vi "turnOppositeToEnemy.vi"(0 "KickToSkill in":refnum<class "KickToSkill.lvclass">, 5 "BallRef":refnum<class "Ball.lvclass">, 7 "Robot":refnum<class "Robot.lvclass">, 9 "EnemyRobotRef":refnum<class "Robot.lvclass">[](array[class]), 11 "error in (no error)":errorcluster) -> (4 "KickToSkill out":refnum<class "KickToSkill.lvclass">, 6 "state out":T1=enum."Farthest", 15 "error out":errorcluster)   [LabVIEW 2020, in "KickToSkill.lvclass"]
uses:
  KickToSkill.lvclass
  Robot_class/Robot.lvclass
  C:/Users/anton/Desktop/RoboIME/SSL_COMP/SSL_AI/Object_class/Object.lvclass
  Ball_class/Ball.lvclass
  turnOppositeToEnemyStates.ctl
  Object_class/Object.lvclass/Object.ctl
  Robot_class/Robot.lvclass/Robot.ctl
  <vilib>/Analysis/baseanly.llb/Real Dot Product.vi
  Object_class/Read x.vi
  Object_class/Read y.vi
  Robot_class/Read dest_orientation.vi
  Utilities_class/Utilities.lvclass
  <vilib>/Analysis/NI_AALBase.lvlib
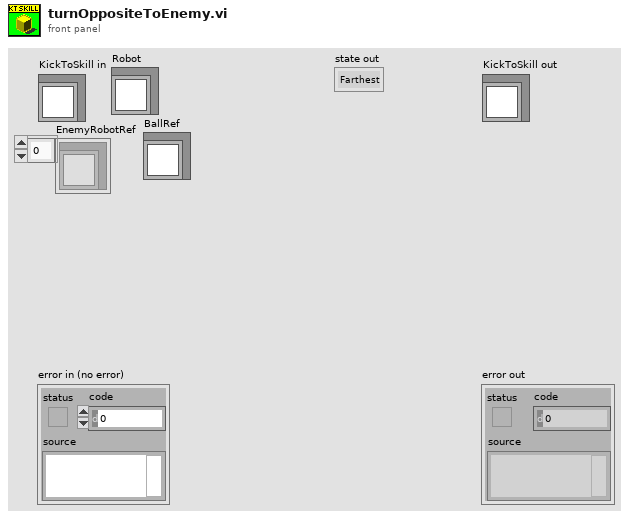
[diagram p1: front panel]
types:
  T1 = typedef "turnOppositeToEnemyStates.ctl" = enum16{"None", "Closest", "Farthest"}
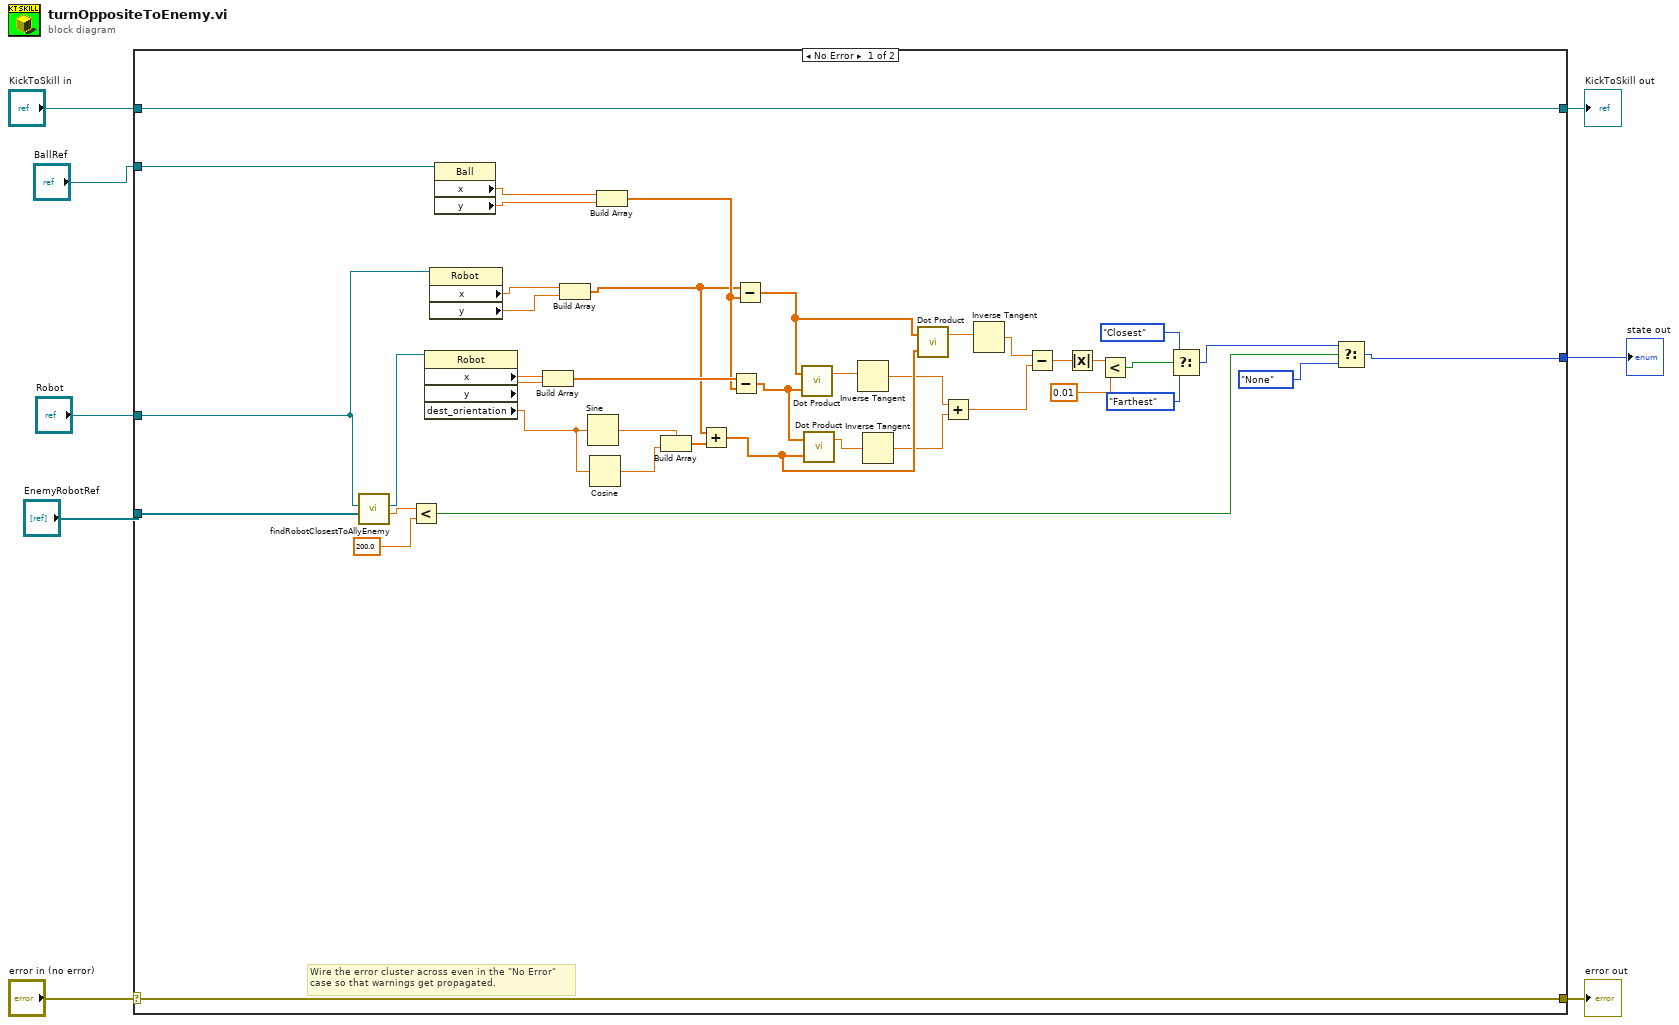
[diagram p0: block diagram]
diagram:
  n1 = case shown="No Error" "error in (no error)" {
    selector: "error in (no error)" -> [w48 w51]
    tunnel: [w48 w51] -> w7
    tunnel: [w49 w50] -> w5
    tunnel: "KickToSkill in" -> [w49 w50]
    tunnel: "EnemyRobotRef" -> [w47 _]
    tunnel: "Robot" -> [w44 _]
    tunnel: "BallRef" -> [w38 _]
    tunnel: [w9 _] -> w1
    frame No Error {
      # "Wire the error cluster across even in the \"No Error\"\ncase so that warnings get propagated."
      n2 = call "findRobotClosestToAllyEnemy.vi"("Ally/Enemy Robots"=w47, "Robot Target"=w44) -> ("Robot distance to other one"=w46:dbl, "Robot"=w43:refnum<class "Robot.lvclass">)  [unwired: 6 in, 2 out]
      n3 = Less?(x=w46, y=200.0 ("Robot distance to other one")) -> (x < y?=w33:bool)
      n4 = property class="Robot"(reference=w43) -> ("x"=w40:dbl, "y"=w39:dbl, "dest_orientation"=w31:dbl)  [unwired: 1 in, 2 out]
      n5 = property class="Robot"(reference=w44) -> ("x"=w42:dbl, "y"=w41:dbl)  [unwired: 1 in, 2 out]
      n6 = property class="Ball"(reference=w38) -> ("x"=w37:dbl, "y"=w36:dbl)  [unwired: 1 in, 2 out]
      n7 = Build Array(w40, w39) -> (w35:dbl[])
      n8 = Build Array(w42, w41) -> (w27:dbl[])
      n9 = Sine(x=w31) -> (sin(x)=w30:dbl)
      n10 = Cosine(x=w31) -> (cos(x)=w29:dbl)
      n11 = Build Array(w37, w36) -> (w34:dbl[])
      n12 = Build Array(w30, w29) -> (w28:dbl[])
      n13 = Add(x=w27, y=w28) -> (x+y=w24:dbl[])
      n14 = Subtract(x=w35, y=w34) -> (x-y=w26:dbl[])
      n15 = Subtract(x=w27, y=w34) -> (x-y=w25:dbl[])
      n16 = call-poly <vilib>:"Dot Product.vi"("Y Vector"=w26, "X Vector"=w25) -> ("X * Y"=w22:dbl)  [unwired: 1 out]
      n17 = call-poly <vilib>:"Dot Product.vi"("Y Vector"=w24, "X Vector"=w26) -> ("X * Y"=w23:dbl)  [unwired: 1 out]
      n18 = Inverse Tangent(1:w22) -> (0:w20:dbl)
      n19 = Inverse Tangent(1:w23) -> (0:w19:dbl)
      n20 = call-poly <vilib>:"Dot Product.vi"("Y Vector"=w24, "X Vector"=w25) -> ("X * Y"=w21:dbl)  [unwired: 1 out]
      n21 = Add(x=w20, y=w19) -> (x+y=w17:dbl)
      n22 = Inverse Tangent(1:w21) -> (0:w18:dbl)
      n23 = Subtract(x=w18, y=w17) -> (x-y=w16:dbl)
      n24 = Absolute Value(x=w16) -> (abs(x)=w15:dbl)
      n25 = Less?(x=w15, y=0.01) -> (x < y?=w13:bool)
      n26 = Select(t=turnOppositeToEnemyStates."Closest", s=w13, f=turnOppositeToEnemyStates."Farthest") -> (s? t:f=w10:T1)
      n27 = Select(t=w10, s=w33, f=turnOppositeToEnemyStates."None") -> (s? t:f=w9:T1)
    }
    frame Error {
    }
  }
  "error out" <- w7
  "KickToSkill out" <- w5
  "state out" <- w1
